vi "Set Caption.vi"(8 "error in":errorcluster, 10 "Icon":string, 11 "Title":string) -> (0 "error out":errorcluster)   [LabVIEW 2014, in "LibSDL2.lvlib"]
uses:
  LibSDL2.lvlib
  DLL/SDL2.dll
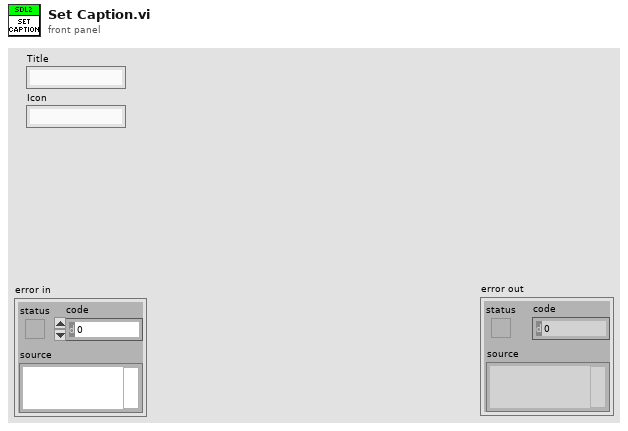
[diagram p1: front panel]
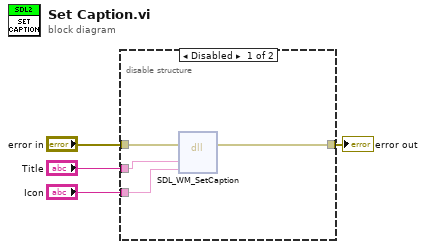
[diagram p0: block diagram]
diagram:
  n1 = disable-structure shown="Disabled" {
    disable-tunnel: "error in" -> [w8 _]
    disable-tunnel: [w7 _] -> w3
    disable-tunnel: "Title" -> [w6 _]
    disable-tunnel: "Icon" -> [w5 _]
    frame Disabled {
      n2 = dll-call lib="C:/dev/PGS/LabSDL2/Source/LibSDL2 Wrapper/DLL/SDL2.dll" fn="SDL_WM_SetCaption"(error in=w8, "file"=w6, "mode"=w5) -> (error out=w7:errorcluster)  [unwired: 5 in, 1 out]
    }
    frame Enabled {
    }
  }
  "error out" <- w3
